vi "pH Gran plot.vi"(4 "accept pH value":bool, 6 "min points":u8=3, 8 "initialize":bool, 9 "amount of titrant added":dbl format="%.2f", 10 "pH":dbl format="%.2f", 11 "sample":T1 {"Nt" format="%.4f"; "Vo" format="%.3f"}) -> (3 "Gran plot":T3={"Ve"=0.5, "ANC"=0.5, "r"=0.5, "Gran type"=enum."ANC", "Gran Plot"=[], "pH"=[]} {"r" format="%.4f"; "ANC" format="%.2p"; "Ve" format="%.3f"; "pH" format="%.2f"})   [LabVIEW 2012]
uses:
  pH Gran plot.ctl
  pH gran type.ctl
  pH titration.ctl
panel:
  # "Normality of titrant"
  # "eq/L"
  # "mL"
  # "Volume of sample"
  # "mL"
  # "eq/L"
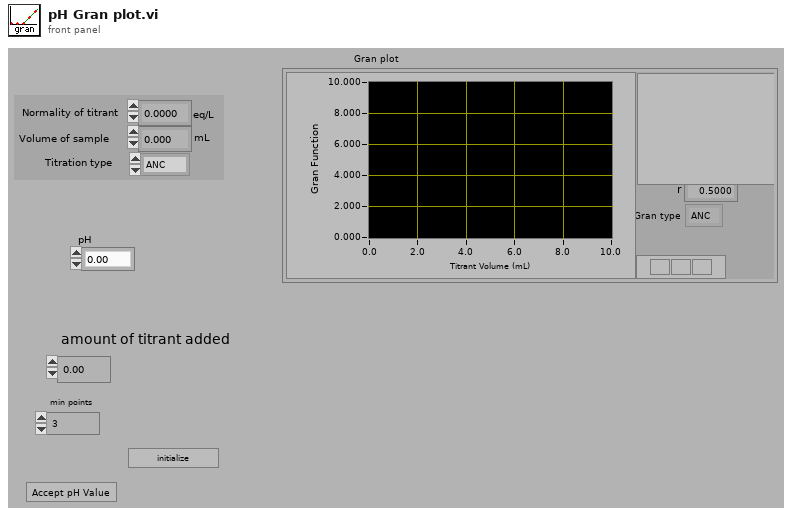
[diagram p1: front panel]
types:
  T1 = typedef "pH titration.ctl" = cluster{"Vo":dbl, "Nt":dbl, "Titration type":T2}
  T2 = typedef "pH gran type.ctl" = enum16{"ANC", "BNC"}
  T3 = typedef "pH Gran plot.ctl" = cluster{"Ve":dbl, "ANC":dbl, "r":dbl, "Gran type":T2, "Gran Plot":cluster{"Va":dbl[], "F1":dbl[]}[], "pH":dbl[]}
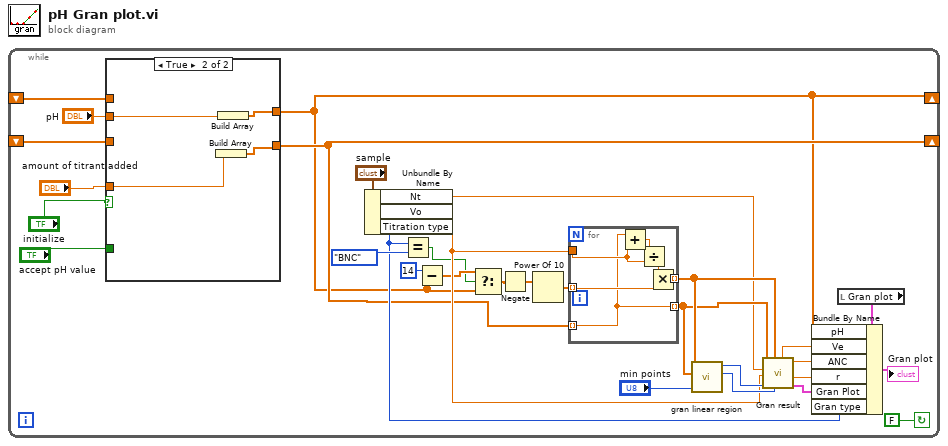
[diagram p0: block diagram]
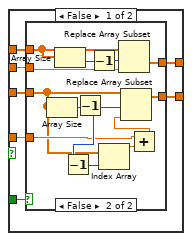
[diagram p2: hidden frame]
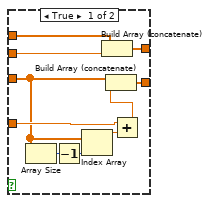
[diagram p3: hidden frame]
diagram:
  n1 = while {
    shift-right: [w3] -> _
    shift-left: _ -> [w7]
    shift-right: [w5] -> _
    shift-left: _ -> [w6]
    stop <- FALSE continue-if-true
    n2 = case shown="True" "initialize" {
      tunnel: "pH" -> [w37 w65]
      tunnel: "amount of titrant added" -> [w33 w64]
      tunnel: [w36 w63] -> w3
      tunnel: w7 -> [w38 _]
      tunnel: [w35 w62] -> w5
      tunnel: w6 -> [w34 _]
      tunnel: "accept pH value" -> [w32 _]
      frame False {
        n3 = case shown="False" w32 {
          tunnel: w38 -> [w40 w54]
          tunnel: w37 -> [w48 w56]
          tunnel: [w47 w55] -> w36
          tunnel: [w46 w51] -> w35
          tunnel: w34 -> [w39 w50]
          tunnel: w33 -> [w42 w58]
          frame True {
            n4 = Array Size(array=w39) -> (size(s)=w43:i32)
            n5 = Decrement(x=w43) -> (x-1=w44:i32)
            n6 = Index Array(array=w39, index=w44) -> (element=w45:dbl)
            n7 = Build Array (concatenate)(w40, w48) -> (w47:dbl[])
            n8 = Add(x=w42, y=w45) -> (x+y=w41:dbl)
            n9 = Build Array (concatenate)(w39, w41) -> (w46:dbl[])
          }
          frame False {
            n10 = Array Size(array=w50) -> (size(s)=w59:i32)
            n11 = Array Size(array=w54) -> (size(s)=w53:i32)
            n12 = Decrement(x=w59) -> (x-1=w60:i32)
            n13 = Decrement(x=w60) -> (x-1=w49:i32)
            n14 = Decrement(x=w53) -> (x-1=w52:i32)
            n15 = Index Array(array=w50, index=w49) -> (element=w61:dbl)
            n16 = Replace Array Subset(array=w54, new element=w56, index=w52) -> (w55:dbl[])
            n17 = Add(x=w58, y=w61) -> (x+y=w57:dbl)
            n18 = Replace Array Subset(array=w50, new element=w57, index=w60) -> (w51:dbl[])
          }
        }
      }
      frame True {
        n19 = Build Array(w64) -> (w62:dbl[])
        n20 = Build Array(w65) -> (w63:dbl[])
      }
    }
    n21 = Unbundle By Name("sample") -> ("Nt"=w22:dbl, "Vo"=w23:dbl, "Titration type"=w12:T2)
    n22 = Equal?(x=w12, y=pH_gran_type."BNC" ("Titration type")) -> (x = y?=w16:bool)
    n23 = Subtract(x=14, y=w3) -> (x-y=w18:dbl[])
    n24 = Select(t=w18, s=w16, f=w3) -> (s? t:f=w21:dbl[])
    n25 = Negate(x=w21) -> (-x=w20:dbl[])
    n26 = Power Of 10(x=w20) -> (10^x=w31:dbl[])
    n27 = for {
      tunnel: w31 -> [w70] mode=indexing
      tunnel: [w67] -> w29 mode=indexing
      tunnel: w5 -> [w66] mode=indexing
      tunnel: w23 -> [w68]
      tunnel: [w66] -> w28 mode=indexing
      n28 = Add(x=w66, y=w68) -> (x+y=w71:dbl)
      n29 = Divide(x=w71, y=w68) -> (x/y=w69:dbl)
      n30 = Multiply(x=w69, y=w70) -> (x*y=w67:dbl)
    }
    n31 = call "gran linear region.vi"("min points"="min points", "Va"=w28, "F1"=w29) -> ("first i"=w26:u8, "length"=w27:u8)  [unwired: 7 in]
    n32 = call "Gran result.vi"("first i"=w26, "F1"=w29, "length"=w27, "Vo"=w23, "Nt"=w22, "Vt"=w28) -> ("graph"=w10:cluster{"Vt":dbl[], "F1":dbl[]}[], "r"=w13:dbl, "ANC"=w14:dbl, "Ve"=w15:dbl)  [unwired: 1 in, 1 out]
    n33 = local read "Gran plot"() -> (w30:T3)
    n34 = Bundle By Name(cluster=w30, "pH"=w3, "Ve"=w15, "ANC"=w14, "r"=w13, "Gran Plot"=w10, "Gran type"=w12) -> (→"Gran plot":T3)
  }
